vi "GetCalInj.vi"(7 "LabVIEW Web Service Request":refnum<class "Web Request.lvclass">) -> (3 "CalInj":string)   [LabVIEW 2016]
uses:
  <vilib>/wsapi/Web Request.lvclass
  controls/MotorStates.ctl
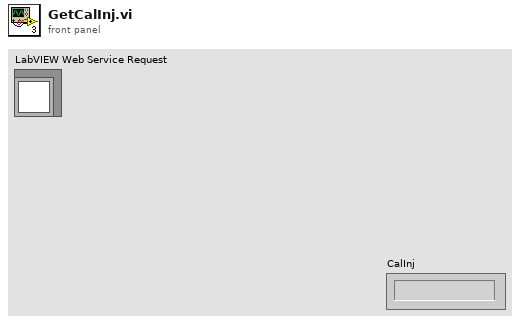
[diagram p1: front panel]
types:
  T1 = typedef "RT-Variables.lvlib/MotorStates.ctl" = enum16{"Open", "Close", "Moving", "Screwed"}
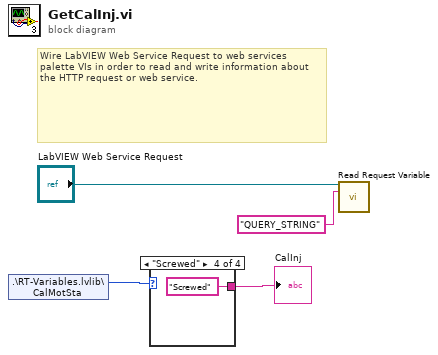
[diagram p0: block diagram]
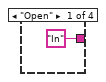
[diagram p2: hidden frame]
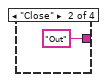
[diagram p3: hidden frame]
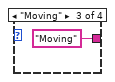
[diagram p4: hidden frame]
diagram:
  # "Wire LabVIEW Web Service Request to web services palette VIs in order to read and write information about the HTTP request or web service."
  n1 = shared-variable ".\\RT-Variables.lvlib\\CalMotSta"() -> (w1:T1)  [unwired: 1 in, 1 out]
  n2 = case shown="\"Screwed\"" w1 {
    tunnel: ["In" ("EnvCover") "Out" ("EnvCover") "Moving" ("EnvCover") "Screwed" ("EnvCover")] -> w2
    frame "Open" {
    }
    frame "Close" {
    }
    frame "Moving" {
    }
    frame "Screwed" {
    }
  }
  "CalInj" <- w2
  n3 = call <vilib>:"Read Request Variable.vi"("LabVIEW Web Service Request"="LabVIEW Web Service Request", "variable name"="QUERY_STRING") -> ()  [unwired: 11 in, 3 out]
